vi "Timer.vi"(8 "error in (no error)":errorcluster, 10 "Time Target (s)":dbl=60.0 format="%#_13g", 11 "Timer Action":string(combo)) -> (0 "error out":errorcluster, 2 "Time has Elapsed":bool, 3 "Present (s)":dbl)   [LabVIEW 2021]
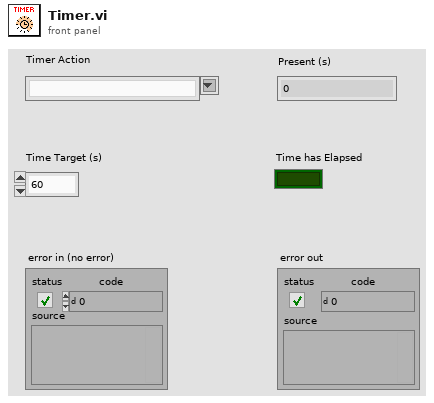
[diagram p1: front panel]
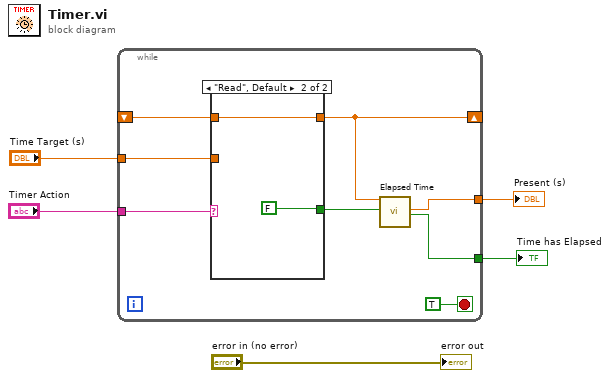
[diagram p0: block diagram]
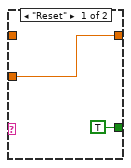
[diagram p2: hidden frame]
diagram:
  n1 = while {
    tunnel: "Timer Action" -> [w13]
    tunnel: [w6] -> w4
    tunnel: [w12] -> w3
    shift-right: [w7] -> _
    shift-left: _ -> [w9]
    tunnel: "Time Target (s)" -> [w8]
    stop <- TRUE stop-if-true
    n2 = case shown="\"Read\", Default" w13 {
      tunnel: [TRUE FALSE] -> w11
      tunnel: w8 -> [w14 _]
      tunnel: w9 -> [_ w16]
      tunnel: [w14 w16] -> w7
      frame "Reset" {
      }
      frame "Read", Default {
      }
    }
    n3 = call "Elapsed Time"("Time Target (s)"=w7, "Reset"=w11) -> ("Elapsed Time (s)"=w6:dbl, "Time has Elapsed"=w12:bool)  [unwired: 10 in, 6 out]
  }
  "Present (s)" <- w4
  "Time has Elapsed" <- w3
  "error out" <- "error in (no error)"
